vi "UT_010_TOML to LV_enum.vi"() -> ()   [LabVIEW 2017]
uses:
  a84c01b4-b6b6-4be3-a592-8d4feadcdc62.vi
  8d36a4aa-f2c5-4afc-9410-2bff02845cb1.vi
  lib/TOML to LabVIEW.vi
  <vilib>/addons/_JKI Toolkits/Caraya/classes/Assert/Assert Equal Value_Variant.vi
  <vilib>/addons/_JKI Toolkits/Caraya/classes/Assert/Assert Error.vi
  <vilib>/addons/_JKI Toolkits/Caraya/classes/Test/Test.lvclass
  <vilib>/addons/_JKI Toolkits/Caraya/classes/Assert/Assert.lvclass
  lib/TOML.lvlib
panel:
  out "error out":errorcluster
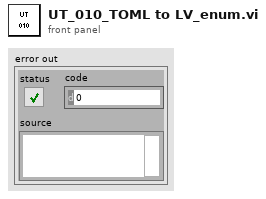
[diagram p1: front panel]
types:
  T1 = cluster{"cluster":cluster{"enum":enum16{"false", "true"}}}
  T2 = typedef "TOML.lvlib/TOML Value.ctl" = cluster{"type":enum16{"Table", "Array", "String", "Integer", "Float", "Boolean", "Offset Date-Time", "Local Date-Time", "Local Date", "Local Time", "Path"}, "value":variant}
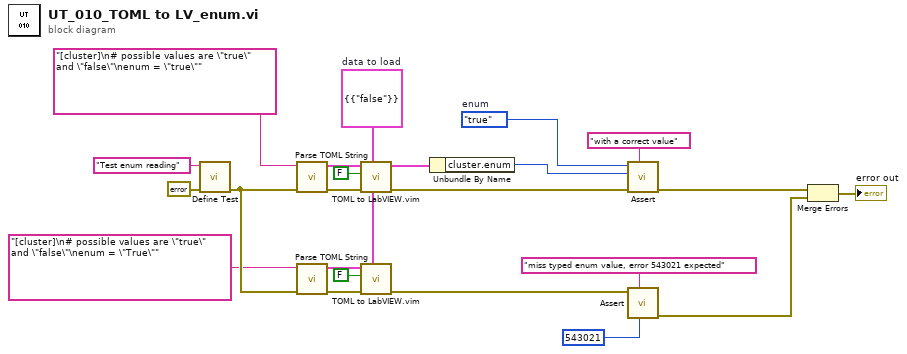
[diagram p0: block diagram]
diagram:
  w3 = enum16{"false", "true"}."true"  # enum
  w5 = T1 {"cluster"={"enum"=enum."false"}}  # data to load
  n1 = call <vilib>:"Define Test.vi"("error in (no error)"=errorcluster {"status"=FALSE, "code"=0, "source"=""}, "Label (VI Title)"="Test enum reading") -> ("error out"=w16:errorcluster)  [unwired: 9 in]
  n2 = call "Parse TOML String.vi"("error in (no error)"=w16, "String"="[cluster]\n# possible values are \"true\" and \"false\"\nenum = \"true\"") -> ("error out"=w13:errorcluster, "Value"=w14:T2)  [unwired: 8 in]
  n3 = call "Parse TOML String.vi"("error in (no error)"=w16, "String"="[cluster]\n# possible values are \"true\" and \"false\"\nenum = \"True\"") -> ("error out"=w8:errorcluster, "Value"=w10:T2)  [unwired: 8 in]
  n4 = call "TOML to LabVIEW.vim"("datatype"=w5, "error in (no error)"=w13, "Error if missing element"=FALSE, "Value"=w14) -> ("error out"=w12:errorcluster, "LV Data"=w7:T1)  [unwired: 5 in, 1 out]
  n5 = call "TOML to LabVIEW.vim"("datatype"=w5, "error in (no error)"=w8, "Error if missing element"=FALSE, "Value"=w10) -> ("error out"=w1:errorcluster)  [unwired: 5 in, 2 out]
  n6 = Unbundle By Name(w7) -> ("cluster.enum"=w6:enum16{"false", "true"})
  n7 = call-poly <vilib>:"Assert.vi"("Label"="with a correct value" ("Label (VI Title)"), "error in (no error)"=w12, "Y"=w6, "X"=w3) -> ("error out"=w22:errorcluster)  [unwired: 7 in]
  n8 = call-poly <vilib>:"Assert.vi"("error code (1)"=543021, "Label"="miss typed enum value, error 543021 expected" ("Label (VI Title)"), "Error?"=w1) -> ("error out"=w17:errorcluster)  [unwired: 8 in]
  n9 = Merge Errors(w22, w17) -> (→"error out":errorcluster)
